vi "Close.vi"(8 "error in (no error)":errorcluster, 11 "CIPC Reference":u64) -> (0 "error out":errorcluster)   [LabVIEW 2021, in "CIF_NI_CIPC.lvlib"]
doc: "Close the reference to the buffer without destroying the buffer."
uses:
  CIF_NI_CIPC.lvlib
  <vilib>/Utility/error.llb/Trim Whitespace.vi
  <vilib>/Utility/error.llb/Error Cluster From Error Code.vi
  libnicipc.dll
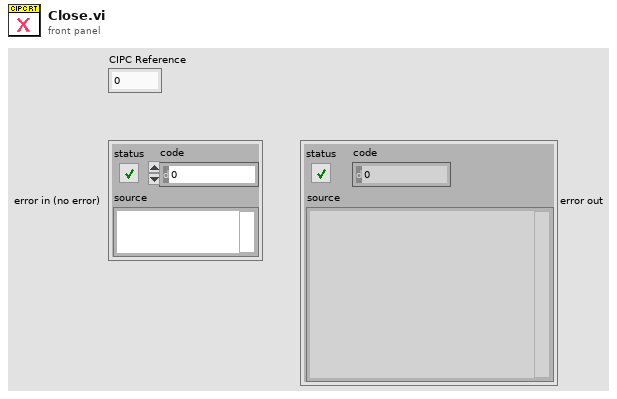
[diagram p1: front panel]
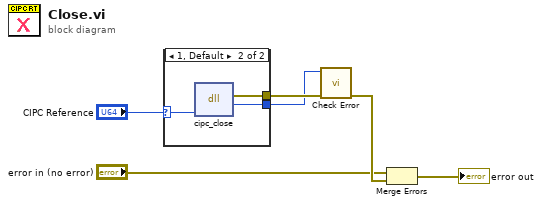
[diagram p0: block diagram]
diagram:
  n1 = case shown="1, Default" "CIPC Reference" {
    selector: "CIPC Reference" -> [_ w7]
    tunnel: [_ w9] -> w6
    tunnel: [_ w8] -> w5
    frame 0 {
    }
    frame 1, Default {
      n2 = dll-call lib="libnicipc.*" fn="cipc_close"("cipc_buffer_ref"=w7) -> (error out=w9:errorcluster, "return type"=w8:i32)  [unwired: 4 in, 1 out]
    }
  }
  n3 = call "Check Error.vi"("error in (no error)"=w6, "Error Code"=w5) -> ("error out"=w4:errorcluster)  [unwired: 9 in]
  n4 = Merge Errors("error in (no error)", w4) -> (→"error out":errorcluster)
